vi "gen_multi_trace_file_paths.vi"(7 "Generic trace file path":path) -> (4 "avg_IR_off_path":path, 8 "avg_IR_on_path":path, 13 "avg_IR_power_path":path, 15 "avg_diff_path":path)   [LabVIEW 2020]
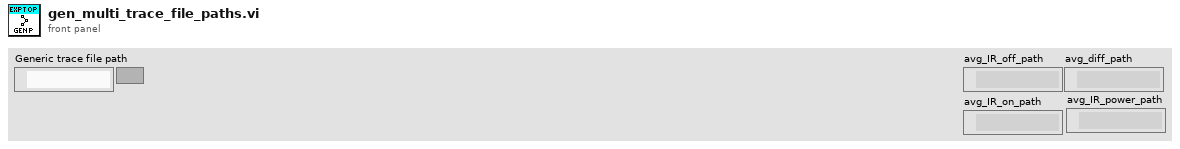
[diagram p1: front panel]
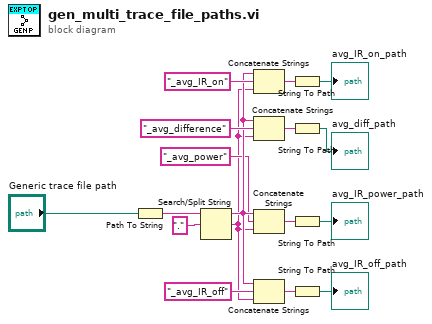
[diagram p0: block diagram]
diagram:
  n1 = Path To String(path="Generic trace file path") -> (string=w16:string)
  n2 = Search/Split String(string=w16, search string/char (-)=".") -> (substring before match=w5:string, match + rest of string=w3:string)  [unwired: 1 in, 1 out]
  n3 = Concatenate Strings(w5, "_avg_IR_on" ("string"), w3) -> (w10:string)
  n4 = Concatenate Strings(w5, "_avg_difference" ("string"), w3) -> (w9:string)
  n5 = Concatenate Strings(w5, "_avg_power" ("string"), w3) -> (w2:string)
  n6 = Concatenate Strings(w5, "_avg_IR_off" ("string"), w3) -> (w11:string)
  n7 = String To Path(string=w10) -> (path=→"avg_IR_on_path":path)
  n8 = String To Path(string=w9) -> (path=→"avg_diff_path":path)
  n9 = String To Path(string=w2) -> (path=→"avg_IR_power_path":path)
  n10 = String To Path(string=w11) -> (path=→"avg_IR_off_path":path)
